vi "S2C_M2p5942_Proc_ResetCtrls.vi"(8 "Error In":errorcluster, 11 "Data":T1) -> (0 "Error Out":errorcluster)   [LabVIEW 2015]
uses:
  S2C_M2p5942_Proc_Globals.vi
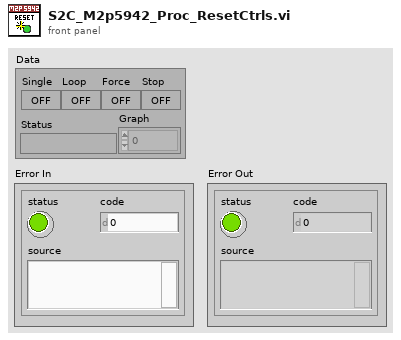
[diagram p1: front panel]
types:
  T1 = cluster{"Single":bool, "Loop":bool, "Force":bool, "Status":string, "Stop":bool, "Graph":sgl[][]}
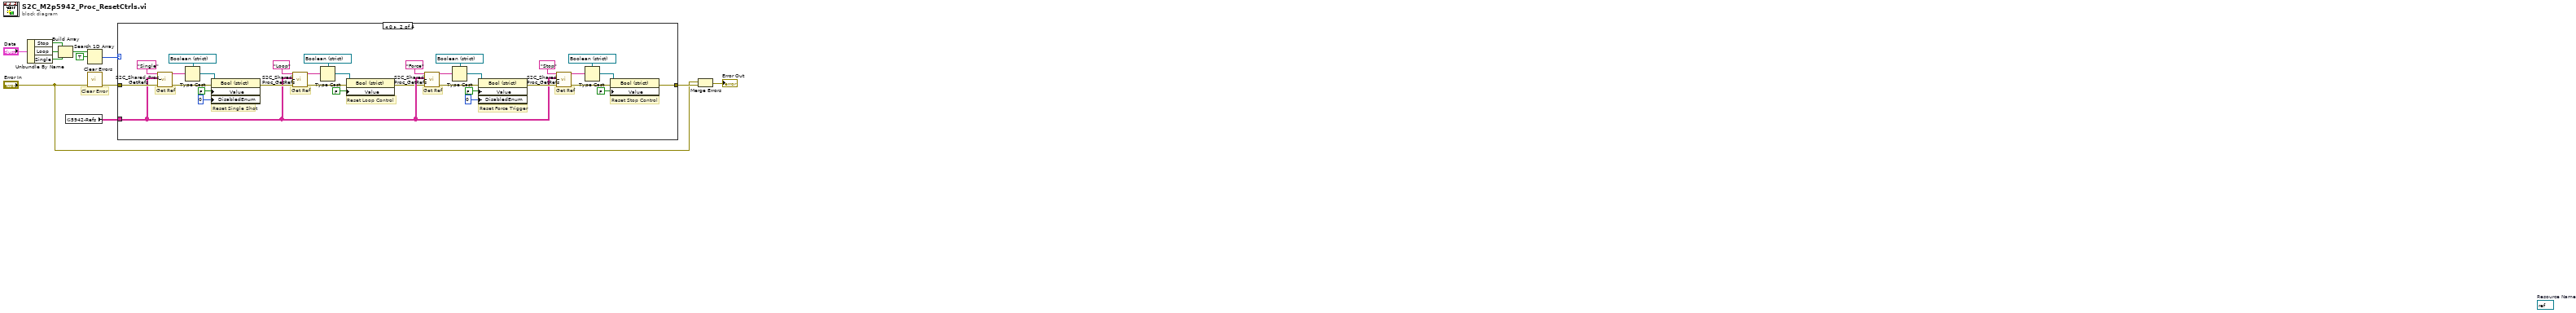
[diagram p0: block diagram]
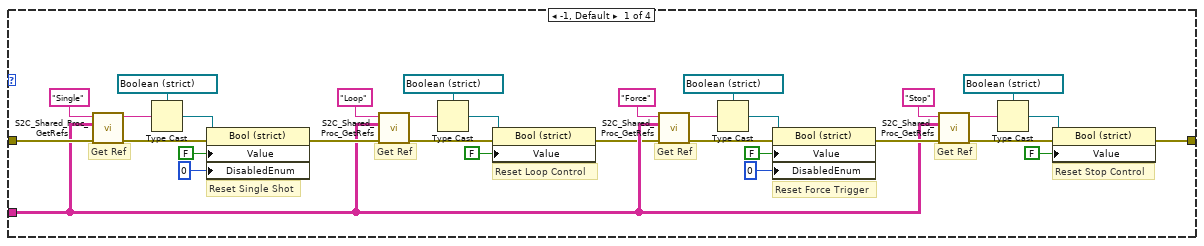
[diagram p2: hidden frame]
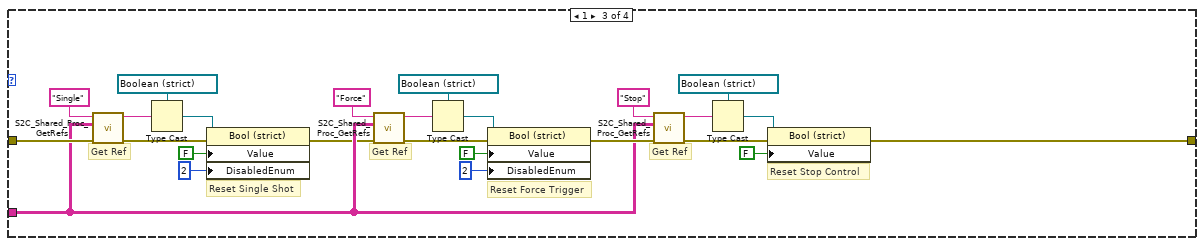
[diagram p3: hidden frame]
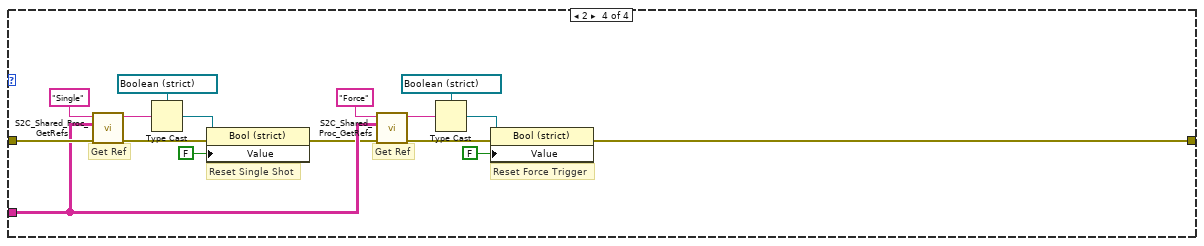
[diagram p4: hidden frame]
diagram:
  (unwired) refnum<visa-resource-name> refnum  # Resource Name
  # "Clear Error"
  n1 = Unbundle By Name("Data") -> ("Stop"=w9:bool, "Loop"=w10:bool, "Single"=w8:bool)
  n2 = Build Array(w9, w10, w8) -> (w7:bool[])
  n3 = global read "S2C_M2p5942_Proc_Globals.vi" "5942-Refs"() -> (w11:string[][])
  n4 = Search 1D Array(1D array=w7, element=TRUE) -> (index of element=w5:i32)  [unwired: 1 in]
  n5 = call <vilib>:"Clear Errors.vi"("error in (no error)"="Error In") -> ("error out"=w4:errorcluster)  [unwired: 5 in, 1 out]
  n6 = case shown="0" w5 {
    tunnel: w4 -> [w38 w70 w95 w111]
    tunnel: [w24 w56 w81 w102] -> w3
    tunnel: w11 -> [w14 w46 w78 w104]
    frame -1, Default {
      # "Reset Loop Control"
      # "Get Ref"
      # "Reset Stop Control"
      # "Get Ref"
      # "Reset Force Trigger"
      # "Get Ref"
      # "Reset Single Shot"
      # "Get Ref"
      n7 = call "S2C_Shared_Proc_GetRefs.vi"("Error In"=w38, "Refs"=w14, "Label"="Single") -> ("Error Out"=w39:errorcluster, "Reference"=w41:string)  [unwired: 7 in]
      n8 = Type Cast(type=refnum<vi> refnum ("Force Trigger?"), x=w41) -> (*(type *) &x=w40:refnum<vi>)
      n9 = property class="Bool (strict)"(reference=w40, error in=w39, "Value"=FALSE, "DisabledEnum"=u8 0) -> (error out=w15:errorcluster)  [unwired: 1 out]
      n10 = call "S2C_Shared_Proc_GetRefs.vi"("Error In"=w15, "Refs"=w14, "Label"="Loop") -> ("Error Out"=w21:errorcluster, "Reference"=w19:string)  [unwired: 7 in]
      n11 = Type Cast(type=refnum<vi> refnum ("Force Trigger?"), x=w19) -> (*(type *) &x=w20:refnum<vi>)
      n12 = property class="Bool (strict)"(reference=w20, error in=w21, "Value"=FALSE) -> (error out=w13:errorcluster)  [unwired: 1 out]
      n13 = call "S2C_Shared_Proc_GetRefs.vi"("Error In"=w13, "Refs"=w14, "Label"="Force") -> ("Error Out"=w37:errorcluster, "Reference"=w35:string)  [unwired: 7 in]
      n14 = Type Cast(type=refnum<vi> refnum ("Force Trigger?"), x=w35) -> (*(type *) &x=w36:refnum<vi>)
      n15 = property class="Bool (strict)"(reference=w36, error in=w37, "Value"=FALSE, "DisabledEnum"=u8 0) -> (error out=w25:errorcluster)  [unwired: 1 out]
      n16 = call "S2C_Shared_Proc_GetRefs.vi"("Error In"=w25, "Refs"=w14, "Label"="Stop") -> ("Error Out"=w26:errorcluster, "Reference"=w28:string)  [unwired: 7 in]
      n17 = Type Cast(type=refnum<vi> refnum ("Force Trigger?"), x=w28) -> (*(type *) &x=w27:refnum<vi>)
      n18 = property class="Bool (strict)"(reference=w27, error in=w26, "Value"=FALSE) -> (error out=w24:errorcluster)  [unwired: 1 out]
    }
    frame 0 {
      # "Reset Loop Control"
      # "Get Ref"
      # "Reset Stop Control"
      # "Get Ref"
      # "Reset Force Trigger"
      # "Get Ref"
      # "Reset Single Shot"
      # "Get Ref"
      n19 = call "S2C_Shared_Proc_GetRefs.vi"("Error In"=w70, "Refs"=w46, "Label"="Single") -> ("Error Out"=w71:errorcluster, "Reference"=w73:string)  [unwired: 7 in]
      n20 = Type Cast(type=refnum<vi> refnum ("Force Trigger?"), x=w73) -> (*(type *) &x=w72:refnum<vi>)
      n21 = property class="Bool (strict)"(reference=w72, error in=w71, "Value"=FALSE, "DisabledEnum"=u8 0) -> (error out=w47:errorcluster)  [unwired: 1 out]
      n22 = call "S2C_Shared_Proc_GetRefs.vi"("Error In"=w47, "Refs"=w46, "Label"="Loop") -> ("Error Out"=w53:errorcluster, "Reference"=w51:string)  [unwired: 7 in]
      n23 = Type Cast(type=refnum<vi> refnum ("Force Trigger?"), x=w51) -> (*(type *) &x=w52:refnum<vi>)
      n24 = property class="Bool (strict)"(reference=w52, error in=w53, "Value"=FALSE) -> (error out=w45:errorcluster)  [unwired: 1 out]
      n25 = call "S2C_Shared_Proc_GetRefs.vi"("Error In"=w45, "Refs"=w46, "Label"="Force") -> ("Error Out"=w69:errorcluster, "Reference"=w67:string)  [unwired: 7 in]
      n26 = Type Cast(type=refnum<vi> refnum ("Force Trigger?"), x=w67) -> (*(type *) &x=w68:refnum<vi>)
      n27 = property class="Bool (strict)"(reference=w68, error in=w69, "Value"=FALSE, "DisabledEnum"=u8 0) -> (error out=w57:errorcluster)  [unwired: 1 out]
      n28 = call "S2C_Shared_Proc_GetRefs.vi"("Error In"=w57, "Refs"=w46, "Label"="Stop") -> ("Error Out"=w58:errorcluster, "Reference"=w60:string)  [unwired: 7 in]
      n29 = Type Cast(type=refnum<vi> refnum ("Force Trigger?"), x=w60) -> (*(type *) &x=w59:refnum<vi>)
      n30 = property class="Bool (strict)"(reference=w59, error in=w58, "Value"=FALSE) -> (error out=w56:errorcluster)  [unwired: 1 out]
    }
    frame 1 {
      # "Reset Stop Control"
      # "Get Ref"
      # "Reset Force Trigger"
      # "Get Ref"
      # "Reset Single Shot"
      # "Get Ref"
      n31 = call "S2C_Shared_Proc_GetRefs.vi"("Error In"=w95, "Refs"=w78, "Label"="Single") -> ("Error Out"=w96:errorcluster, "Reference"=w98:string)  [unwired: 7 in]
      n32 = Type Cast(type=refnum<vi> refnum ("Force Trigger?"), x=w98) -> (*(type *) &x=w97:refnum<vi>)
      n33 = property class="Bool (strict)"(reference=w97, error in=w96, "Value"=FALSE, "DisabledEnum"=u8 2) -> (error out=w77:errorcluster)  [unwired: 1 out]
      n34 = call "S2C_Shared_Proc_GetRefs.vi"("Error In"=w77, "Refs"=w78, "Label"="Force") -> ("Error Out"=w94:errorcluster, "Reference"=w92:string)  [unwired: 7 in]
      n35 = Type Cast(type=refnum<vi> refnum ("Force Trigger?"), x=w92) -> (*(type *) &x=w93:refnum<vi>)
      n36 = property class="Bool (strict)"(reference=w93, error in=w94, "Value"=FALSE, "DisabledEnum"=u8 2) -> (error out=w82:errorcluster)  [unwired: 1 out]
      n37 = call "S2C_Shared_Proc_GetRefs.vi"("Error In"=w82, "Refs"=w78, "Label"="Stop") -> ("Error Out"=w83:errorcluster, "Reference"=w85:string)  [unwired: 7 in]
      n38 = Type Cast(type=refnum<vi> refnum ("Force Trigger?"), x=w85) -> (*(type *) &x=w84:refnum<vi>)
      n39 = property class="Bool (strict)"(reference=w84, error in=w83, "Value"=FALSE) -> (error out=w81:errorcluster)  [unwired: 1 out]
    }
    frame 2 {
      # "Reset Force Trigger"
      # "Get Ref"
      # "Reset Single Shot"
      # "Get Ref"
      n40 = call "S2C_Shared_Proc_GetRefs.vi"("Error In"=w111, "Refs"=w104, "Label"="Single") -> ("Error Out"=w112:errorcluster, "Reference"=w114:string)  [unwired: 7 in]
      n41 = Type Cast(type=refnum<vi> refnum ("Force Trigger?"), x=w114) -> (*(type *) &x=w113:refnum<vi>)
      n42 = property class="Bool (strict)"(reference=w113, error in=w112, "Value"=FALSE) -> (error out=w103:errorcluster)  [unwired: 1 out]
      n43 = call "S2C_Shared_Proc_GetRefs.vi"("Error In"=w103, "Refs"=w104, "Label"="Force") -> ("Error Out"=w110:errorcluster, "Reference"=w108:string)  [unwired: 7 in]
      n44 = Type Cast(type=refnum<vi> refnum ("Force Trigger?"), x=w108) -> (*(type *) &x=w109:refnum<vi>)
      n45 = property class="Bool (strict)"(reference=w109, error in=w110, "Value"=FALSE) -> (error out=w102:errorcluster)  [unwired: 1 out]
    }
  }
  n46 = Merge Errors("Error In", w3) -> (→"Error Out":errorcluster)
